vi "PR4000 cfg mode.vi"(8 "error in (no error)":errorcluster, 10 "Channel parsed command info":T1, 11 "MKS4000b in":refnum<class "MKS4000b.lvclass">) -> (0 "error out":errorcluster, 3 "MKS4000b out":refnum<class "MKS4000b.lvclass">)   [LabVIEW 2013, in "MKS4000b.lvclass"]
uses:
  MKS4000b.lvclass
  Shared/Device Driver/channel parsed cmd cluster.ctl
  channel_mode_typdef.ctl
  MKS4000b.lvclass/MKS4000b.ctl
  shared/CompressAndUpdate(Poly)/CompressAndUpdate(Enum).vi
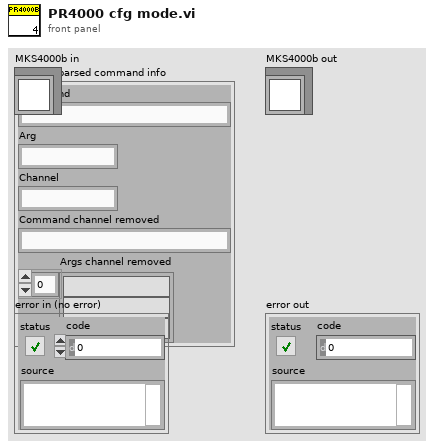
[diagram p1: front panel]
types:
  T1 = typedef "channel parsed cmd cluster.ctl" = cluster{"Command":string, "Arg":string, "Channel":string, "Command channel removed":string, "Args channel removed":string[]}
  T2 = typedef "channel_mode_typdef.ctl" = enum16{"Pressure", "Flow"}
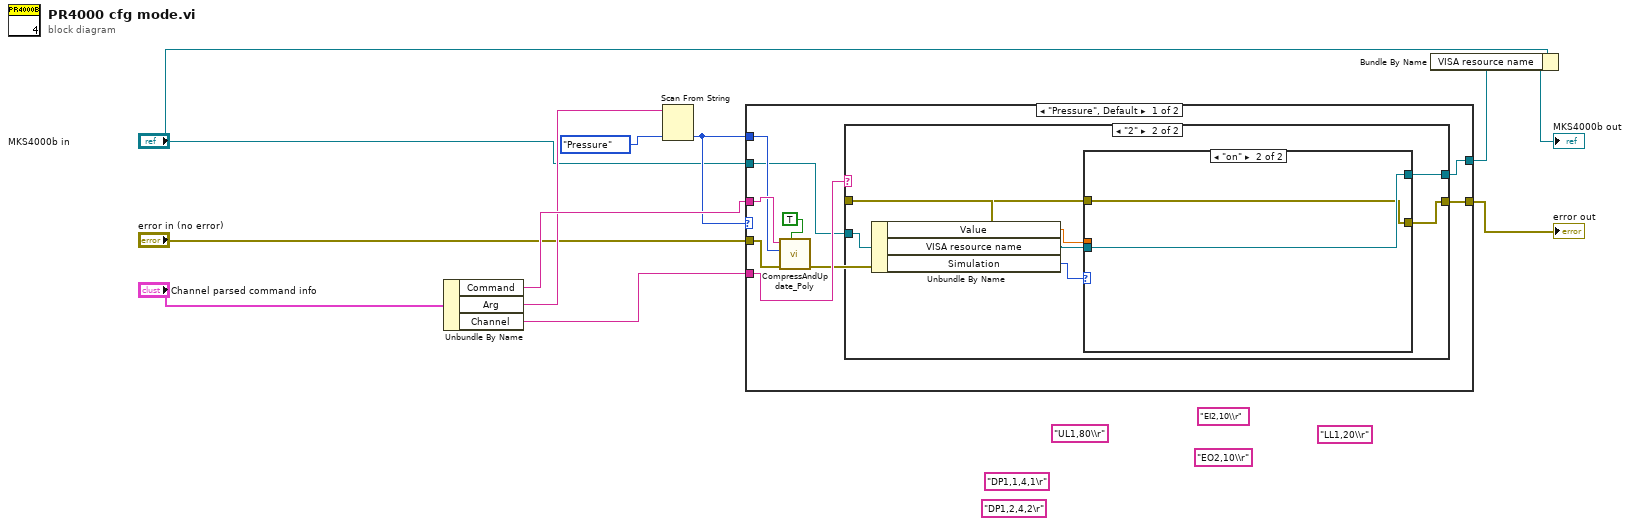
[diagram p0: block diagram]
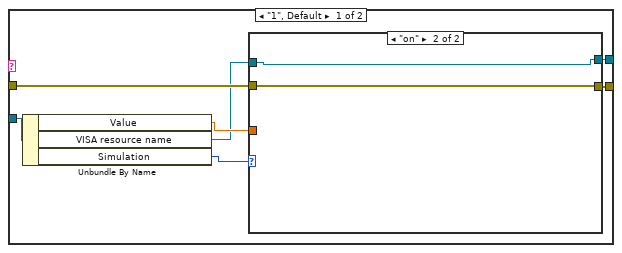
[diagram p2: hidden frame]
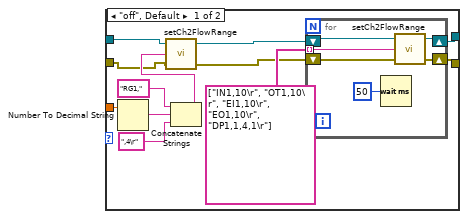
[diagram p3: hidden frame]
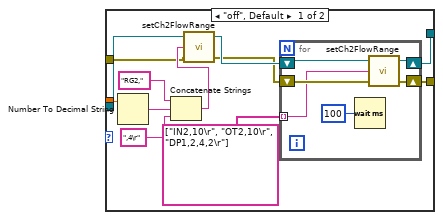
[diagram p4: hidden frame]
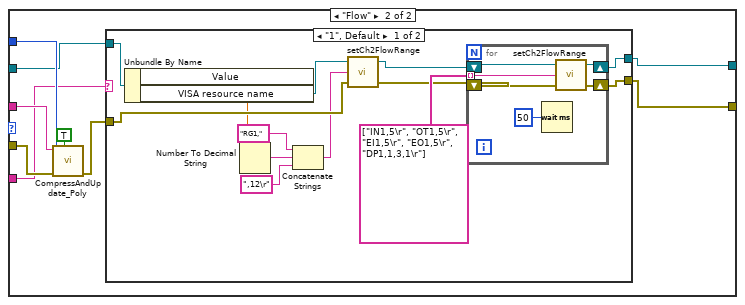
[diagram p5: hidden frame]
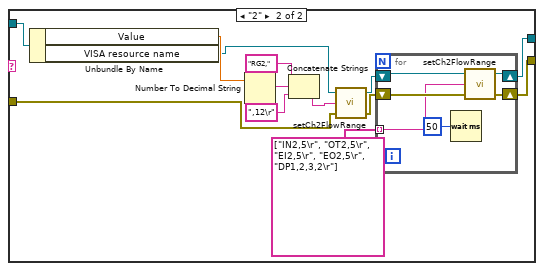
[diagram p6: hidden frame]
diagram:
  (unwired) "DP1,2,4,2\r" ("command in")
  (unwired) "DP1,1,4,1\r" ("command in")
  (unwired) "UL1,80\\r" ("command in")
  (unwired) "LL1,20\\r" ("command in")
  (unwired) "EO2,10\\r" ("command in")
  (unwired) "EI2,10\\r" ("command in")
  n1 = Unbundle By Name("Channel parsed command info") -> ("Command"=w11:string, "Arg"=w10:string, "Channel"=w9:string)
  n2 = Scan From String(input string=w10, default 1=channel_mode_typdef."Pressure" ("Channel 1")) -> (output 1=w6:T2)  [unwired: 3 in, 3 out]
  n3 = case shown="\"Pressure\", Default" w6 {
    tunnel: "error in (no error)" -> [w15 w82]
    tunnel: "MKS4000b in" -> [w12 w75]
    tunnel: [w19 w76] -> w4
    tunnel: w6 -> [w16 w80]
    tunnel: w11 -> [w17 w79]
    tunnel: w9 -> [w20 w78]
    tunnel: [w18 w77] -> w7
    frame "Pressure", Default {
      n4 = call-poly "CompressAndUpdate_Poly.vi"("force CVT update (false)"=TRUE ("force CVT update"), "error in"=w15, "enum variant"=w16, "command or variable name"=w17) -> ("error out"=w14:errorcluster)  [unwired: 7 in]
      n5 = case shown="\"2\"" w20 {
        tunnel: w14 -> [w27 w54]
        tunnel: [w23 w49] -> w19
        tunnel: [w22 w50] -> w18
        tunnel: w12 -> [w26 w53]
        frame "1", Default {
          n6 = Unbundle By Name(w26) -> ("Value"=w25:dbl, "VISA resource name"=w24:refnum<visa-resource-name>, "Simulation"=w21:enum16{"off", "on"})
          n7 = case shown="\"on\"" w21 {
            tunnel: w27 -> [w36 w46]
            tunnel: w25 -> [w35 _]
            tunnel: w24 -> [w34 w47]
            tunnel: [w29 w46] -> w23
            tunnel: [w28 w47] -> w22
            frame "off", Default {
              n8 = Number To Decimal String(number=w35) -> (decimal integer string=w33:string)  [unwired: 1 in]
              n9 = Concatenate Strings("RG1,", w33, ",4\r" ("write buffer")) -> (w37:string)
              n10 = call "setCh2FlowRange.vi"("error"=w36, "command in"=w37, "Comport PR4000"=w34) -> ("error out"=w30:errorcluster, "VISA resource name out"=w31:refnum<visa-resource-name>)  [unwired: 1 out]
              n11 = for {
                tunnel: string[] ["IN1,10\r", "OT1,10\r", "EI1,10\r", "EO1,10\r", "DP1,1,4,1\r"] -> [w43] mode=indexing
                shift-right: [w42] -> w28
                shift-left: w31 -> [w44]
                shift-right: [w41] -> w29
                shift-left: w30 -> [w45]
                n12 = Wait (ms)(milliseconds to wait=u32 50) -> ()  [unwired: 1 out]
                n13 = call "setCh2FlowRange.vi"("error"=w45, "command in"=w43, "Comport PR4000"=w44) -> ("error out"=w41:errorcluster, "VISA resource name out"=w42:refnum<visa-resource-name>)  [unwired: 1 out]
              }
            }
            frame "on" {
            }
          }
        }
        frame "2" {
          n14 = Unbundle By Name(w53) -> ("Value"=w52:dbl, "VISA resource name"=w51:refnum<visa-resource-name>, "Simulation"=w48:enum16{"off", "on"})
          n15 = case shown="\"on\"" w48 {
            tunnel: w54 -> [w63 w73]
            tunnel: w52 -> [w62 _]
            tunnel: w51 -> [w61 w74]
            tunnel: [w56 w74] -> w50
            tunnel: [w55 w73] -> w49
            frame "off", Default {
              n16 = Number To Decimal String(number=w62) -> (decimal integer string=w60:string)  [unwired: 1 in]
              n17 = Concatenate Strings("RG2,", w60, ",4\r" ("write buffer")) -> (w64:string)
              n18 = call "setCh2FlowRange.vi"("error"=w63, "command in"=w64, "Comport PR4000"=w61) -> ("error out"=w57:errorcluster, "VISA resource name out"=w58:refnum<visa-resource-name>)  [unwired: 1 out]
              n19 = for {
                tunnel: string[] ["IN2,10\r", "OT2,10\r", "DP1,2,4,2\r"] -> [w70] mode=indexing
                shift-right: [w69] -> w56
                shift-left: w58 -> [w71]
                shift-right: [w68] -> w55
                shift-left: w57 -> [w72]
                n20 = Wait (ms)(milliseconds to wait=u32 100) -> ()  [unwired: 1 out]
                n21 = call "setCh2FlowRange.vi"("error"=w72, "command in"=w70, "Comport PR4000"=w71) -> ("error out"=w68:errorcluster, "VISA resource name out"=w69:refnum<visa-resource-name>)  [unwired: 1 out]
              }
            }
            frame "on" {
            }
          }
        }
      }
    }
    frame "Flow" {
      n22 = call-poly "CompressAndUpdate_Poly.vi"("force CVT update (false)"=TRUE ("force CVT update"), "error in"=w82, "enum variant"=w80, "command or variable name"=w79) -> ("error out"=w81:errorcluster)  [unwired: 7 in]
      n23 = case shown="\"1\", Default" w78 {
        tunnel: [w85 w105] -> w77
        tunnel: w81 -> [w96 w112]
        tunnel: [w84 w103] -> w76
        tunnel: w75 -> [w91 w110]
        frame "1", Default {
          n24 = Unbundle By Name(w91) -> ("Value"=w89:dbl, "VISA resource name"=w90:refnum<visa-resource-name>)
          n25 = Number To Decimal String(number=w89) -> (decimal integer string=w94:string)  [unwired: 1 in]
          n26 = Concatenate Strings("RG1,", w94, ",12\r" ("write buffer")) -> (w92:string)
          n27 = call "setCh2FlowRange.vi"("error"=w96, "command in"=w92, "Comport PR4000"=w90) -> ("error out"=w86:errorcluster, "VISA resource name out"=w87:refnum<visa-resource-name>)  [unwired: 1 out]
          n28 = for {
            tunnel: string[] ["IN1,5\r", "OT1,5\r", "EI1,5\r", "EO1,5\r", "DP1,1,3,1\r"] -> [w100] mode=indexing
            shift-right: [w99] -> w85
            shift-left: w87 -> [w101]
            shift-right: [w98] -> w84
            shift-left: w86 -> [w102]
            n29 = Wait (ms)(milliseconds to wait=u32 50) -> ()  [unwired: 1 out]
            n30 = call "setCh2FlowRange.vi"("error"=w102, "command in"=w100, "Comport PR4000"=w101) -> ("error out"=w98:errorcluster, "VISA resource name out"=w99:refnum<visa-resource-name>)  [unwired: 1 out]
          }
        }
        frame "2" {
          n31 = Unbundle By Name(w110) -> ("Value"=w109:dbl, "VISA resource name"=w108:refnum<visa-resource-name>)
          n32 = Number To Decimal String(number=w109) -> (decimal integer string=w115:string)  [unwired: 1 in]
          n33 = Concatenate Strings("RG2,", w115, ",12\r" ("write buffer")) -> (w111:string)
          n34 = call "setCh2FlowRange.vi"("error"=w112, "command in"=w111, "Comport PR4000"=w108) -> ("error out"=w104:errorcluster, "VISA resource name out"=w106:refnum<visa-resource-name>)  [unwired: 1 out]
          n35 = for {
            tunnel: string[] ["IN2,5\r", "OT2,5\r", "EI2,5\r", "EO2,5\r", "DP1,2,3,2\r"] -> [w119] mode=indexing
            shift-right: [w118] -> w105
            shift-left: w106 -> [w120]
            shift-right: [w117] -> w103
            shift-left: w104 -> [w121]
            n36 = Wait (ms)(milliseconds to wait=u32 50) -> ()  [unwired: 1 out]
            n37 = call "setCh2FlowRange.vi"("error"=w121, "command in"=w119, "Comport PR4000"=w120) -> ("error out"=w117:errorcluster, "VISA resource name out"=w118:refnum<visa-resource-name>)  [unwired: 1 out]
          }
        }
      }
    }
  }
  "error out" <- w4
  n38 = Bundle By Name(cluster="MKS4000b in", "VISA resource name"=w7) -> (→"MKS4000b out":refnum<class "MKS4000b.lvclass">)
